vi "Select Timestamp Dialog.vi"(8 "error in (no error)":errorcluster, 10 "Command List":string[](array[string])) -> (0 "error out":errorcluster, 1 "Daily?":bool, 2 "Cancelled?":bool, 3 "Time Stamp out":timestamp, 5 "Command out":string)   [LabVIEW 2020, in "CSM-ScheduledCmdWindow.lvlib"]
uses:
  CSM-ScheduledCmdWindow.lvlib
  <userlib>/NEVSTOP-Programming-Palette/Dialog & Interface/Fit VI window to Visible Content_nevstop.vi
  <userlib>/_NEVSTOP/Communicable State Machine(CSM)/_tool/_ui/csm-ui-support.lvlib
panel:
  in  "Command":string(combo)
  in  "Daily checkbox?":bool
  out "Time Left":string
  in  "OK Button":bool
  in  "Cancel Button":bool
  in  "Time Stamp":timestamp format="%<%.0X %x>T"
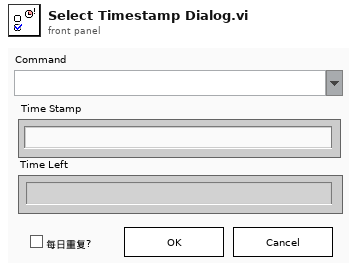
[diagram p1: front panel]
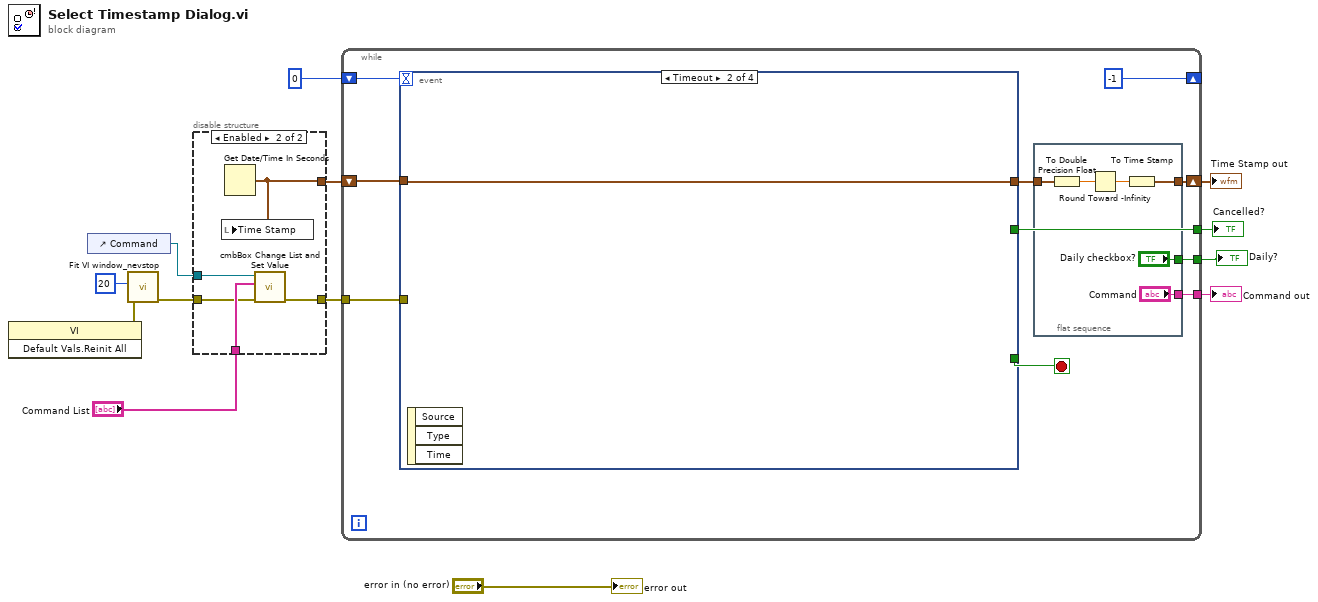
[diagram p0: block diagram]
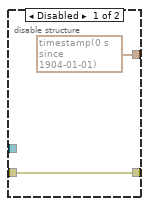
[diagram p2: hidden frame]
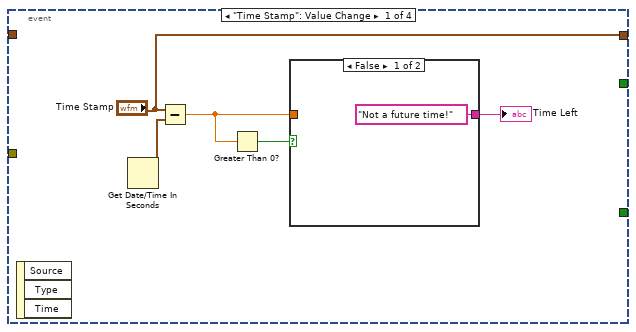
[diagram p3: hidden frame]
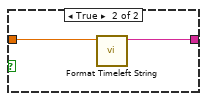
[diagram p4: hidden frame]
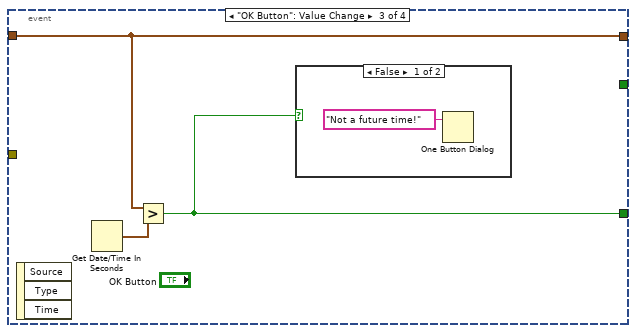
[diagram p5: hidden frame]
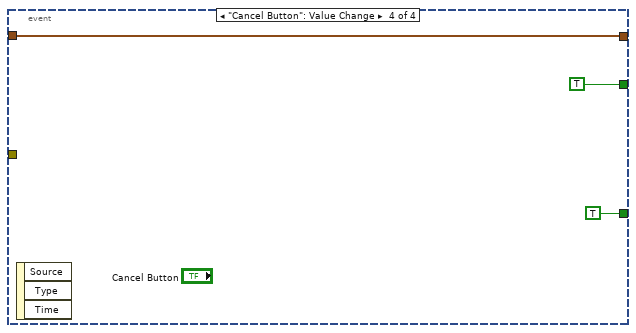
[diagram p7: hidden frame]
diagram:
  n1 = invoke class="VI" method="Default Vals.Reinit All"() -> (error out=w6:errorcluster)  [unwired: 3 in, 2 out]
  n2 = control-ref of="Command"() -> (w2:refnum<vi>)
  n3 = call-poly <userlib>:"Fit VI window_nevstop.vi"("error in (no error)"=w6, "border spacing (2 px)"=20) -> ("error out"=w4:errorcluster)  [unwired: 4 in, 1 out]
  n4 = disable-structure shown="Enabled" {
    disable-tunnel: [timestamp(0 s since 1904-01-01) ("Time Stamp") w20] -> w10
    disable-tunnel: [w14 w17] -> w5
    disable-tunnel: w4 -> [w14 w18]
    disable-tunnel: "Command List" -> [_ w19]
    disable-tunnel: w2 -> [_ w16]
    frame Disabled {
    }
    frame Enabled {
      n5 = Get Date/Time In Seconds() -> (seconds since 1Jan1904=w20:timestamp)
      n6 = local write "Time Stamp"(w20) -> ()
      n7 = call <userlib>:"cmbBox Change List and Set Value.vi"("error in (no error)"=w18, "Strings []"=w19, "cmbBox"=w16) -> ("error out"=w17:errorcluster)  [unwired: 7 in, 1 out]
    }
  }
  n8 = while {
    tunnel: w5 -> [w30]
    shift-right: [w23] -> w9
    shift-left: w10 -> [w29]
    shift-right: [-1] -> _
    shift-left: 0 -> [w28]
    tunnel: [w25] -> w8
    tunnel: [w24] -> w7
    tunnel: [w21] -> w1
    stop <- w26 stop-if-true
    n9 = event shown="[1] Timeout" {
      selector: _ -> [_ _ _ _]
      dyn-events: _ -> [_ _ _ _]
      timeout: w28 -> [_ _ _ _]
      tunnel: w30 -> [_ _ _ _]
      tunnel: ["Time Stamp" w45 w47 w52] -> w22
      tunnel: w29 -> [_ w45 w47 w52]
      tunnel: [_ _ w46 TRUE] -> w26
      tunnel: [_ _ _ TRUE ("Cancelled?")] -> w25
      event "Time Stamp": Value Change {
        n10 = event-data() -> ()  [unwired: 1 in, 3 out]
        n11 = Get Date/Time In Seconds() -> (seconds since 1Jan1904=w40:timestamp)
        n12 = Subtract(x="Time Stamp", y=w40) -> (x-y=w38:dbl)
        n13 = Greater Than 0?(x=w38) -> (x > 0?=w37:bool)
        n14 = case shown="False" w37 {
          tunnel: ["Not a future time!" ("Elapsed Time") w44] -> w41
          tunnel: w38 -> [_ w43]
          frame False {
          }
          frame True {
            n15 = call "Format Timeleft String.vi"("second"=w43) -> ("Elapsed Time"=w44:string)  [unwired: 10 in]
          }
        }
        "Time Left" <- w41
      }
      event Timeout {
        n16 = event-data() -> ()  [unwired: 1 in, 3 out]
      }
      event "OK Button": Value Change {
        n17 = event-data() -> ()  [unwired: 1 in, 3 out]
        n18 = Get Date/Time In Seconds() -> (seconds since 1Jan1904=w48:timestamp)
        n19 = Greater?(x=w47, y=w48) -> (0:w46:bool)
        n20 = case shown="False" w46 {
          frame False {
            n21 = One Button Dialog(message="Not a future time!") -> ()  [unwired: 1 in, 1 out]
          }
          frame True {
          }
        }
      }
      event "Cancel Button": Value Change {
        n22 = event-data() -> ()  [unwired: 1 in, 3 out]
      }
    }
    n23 = flat-sequence {
      tunnel: ["Daily checkbox?"] -> w24
      tunnel: [w32] -> w23
      tunnel: w22 -> [w35]
      tunnel: ["Command"] -> w21
      frame #0 {
        n24 = To Double Precision Float(number=w35) -> (double precision float=w34:dbl)
        n25 = Round Toward -Infinity(1:w34) -> (0:w33:dbl)
        n26 = To Time Stamp(1:w33) -> (0:w32:timestamp)
      }
    }
  }
  "Time Stamp out" <- w9
  "Cancelled?" <- w8
  "Daily?" <- w7
  "Command out" <- w1
  "error out" <- "error in (no error)"
